vi "test Parse Timestamp Array1.vi"(11 "Test Case In":refnum<class "Test Simple CSV Parser.lvclass">) -> (0 "error out":errorcluster, 3 "Test Case Out":refnum<class "Test Simple CSV Parser.lvclass">)   [LabVIEW 2024, in "Test Simple CSV Parser.lvclass"]
uses:
  Test Simple CSV Parser.lvclass
  C:/Program Files/National Instruments/LabVIEW 2025/vi.lib/Astemes/LUnit/Test Case.lvclass
  CSV Parser/Simple CSV Parser/Simple CSV Parser.lvclass
  <vilib>/Astemes/LUnit/Test Case.lvclass/Test Case.ctl
  4993e8ee-a06a-463a-9684-69129f64d5ce.vi
  <vilib>/Astemes/LUnit/Append Pass Result.vi
  <vilib>/Astemes/LUnit/Append Fail Result.vi
  4993e8ee-a06a-463a-9684-69129f64d5ce.vi/9c5d11cd-9439-4240-a1ee-d9baace9c924.vi
  <vilib>/Astemes/LUnit/Run In UI.vi
  <vilib>/Utility/error.llb/Clear Errors.vi
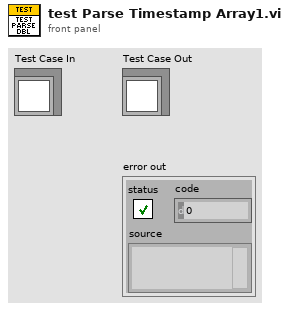
[diagram p1: front panel]
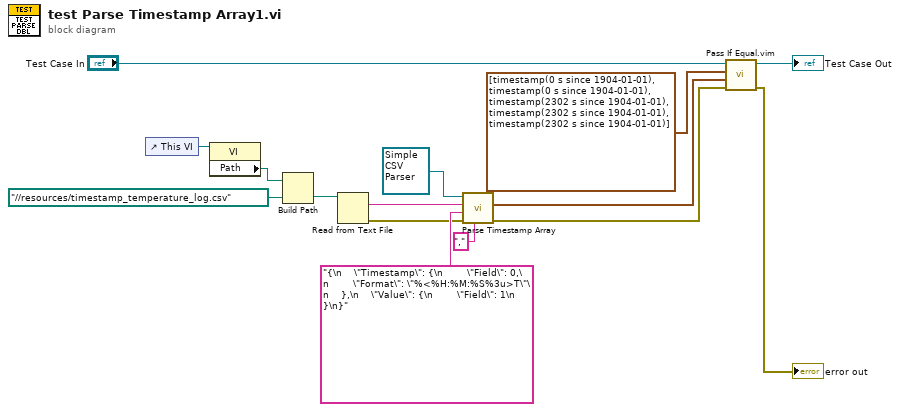
[diagram p0: block diagram]
diagram:
  n1 = control-ref of="This VI"() -> (w9:refnum<vi>)
  n2 = property class="VI"(reference=w9) -> ("Path"=w8:path)  [unwired: 1 in, 2 out]
  n3 = Build Path(base path=w8, name or relative path=path "../../resources/timestamp_temperature_log.csv" ("file (use dialog)")) -> (appended path=w11:path)
  n4 = Read from Text File(file (use dialog)=w11) -> (text=w7:string, error out=w5:errorcluster)  [unwired: 3 in, 2 out]
  n5 = call-dynamic "Parse Timestamp Array.vi"("Seperator"=",", "error in"=w5, "Input <JSON>"="{\n    \"Timestamp\": {\n        \"Field\": 0,\n        \"Format\": \"%<%H:%M:%S%3u>T\"\n    },\n    \"Value\": {\n        \"Field\": 1\n    }\n}", "csv string"=w7, "Simple CSV Parser in"=refnum<class "Simple CSV Parser.lvclass"> refnum) -> ("error out"=w4:errorcluster, "Timestamp Array"=w3:timestamp[])  [unwired: 4 in, 1 out]
  n6 = call "Pass If Equal.vim"("error in (no error)"=w4, "Actual"=w3, "Expected"=timestamp[] [timestamp(0 s since 1904-01-01), timestamp(0 s since 1904-01-01), timestamp(2302.225 s since 1904-01-01), timestamp(2302.325 s since 1904-01-01), timestamp(2302.425 s since 1904-01-01)] ("Timestamp Array"), "LUnit Test Case In"="Test Case In") -> ("error out"=→"error out":errorcluster, "LUnit Test Case Out"=→"Test Case Out":refnum<class "Test Simple CSV Parser.lvclass">)  [unwired: 6 in]
